vi "SPI_Example_Host.vi"() -> ()   [LabVIEW 2012]
uses:
  SPI Host API/Controls/FPGA SPI_SPI Configuration Cluster.ctl
  <vilib>/FPGAPlugInAG/sbRIO-9636/niLvFpga_Open_sbRIO-9636.vi
  <vilib>/FPGAPlugInAG/sbRIO-9636/niLvFpga_Close_sbRIO-9636.vi
  <vilib>/rvi/interface/nirviOpenFPGA/nirviOpenFPGA.xnode
  SPI Host API/Controls/FPGA SPI_FPGA Ref.ctl
  FPGA Bitfiles/NIARC_FPGATarget_SPIFPGATopLevelM_H-QxMroaqT4.lvbitx
  FPGA/SPI_FPGA_Top_Level_Main.vi
  <vilib>/rvi/interface/nirviCloseFPGA/nirviCloseFPGA.xnode
panel:
  out "Byte count":i32
  in  "Perform Startup":bool
  out "array":u8[](array[numeric]) format="%.0x"
  out "error out":errorcluster
  in  "stop":bool
  in  "Write Data":u8[](array[numeric]) format="%.0x"
  in  "Configuration Cluster":T1={"CS"=1, "Clock Rate (Hz)"=50000.0, "Clock Mode"=0, "CS Active State"=FALSE} {"CS" items=["0"=1, "1"=2, "2"=4, "3"=8, "4"=16, "5"=32, "6"=64, "7"=128]; "Clock Mode" items=["0", "1", "2", "3"]}
  in  "Total Bits":u16=8
  out "Read Data":u8[](array[numeric])
  in  "Write":bool
  # "Configure SPI"
  # "Write SPI"
  # "Control and Status"
  # "Read SPI"
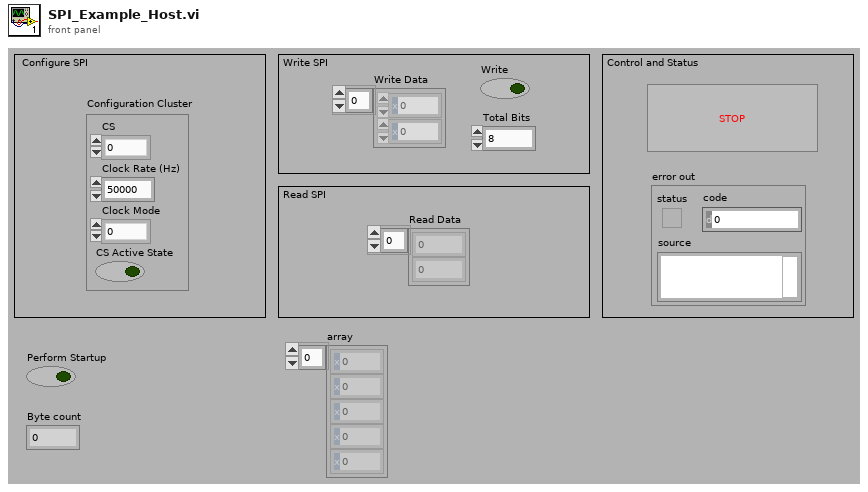
[diagram p1: front panel]
types:
  T1 = typedef "FPGA SPI_SPI Configuration Cluster.ctl" = cluster{"CS":u8, "Clock Rate (Hz)":dbl, "Clock Mode":u8, "CS Active State":bool}
  T2 = typedef "FPGA SPI_FPGA Ref.ctl" = refnum<k20>
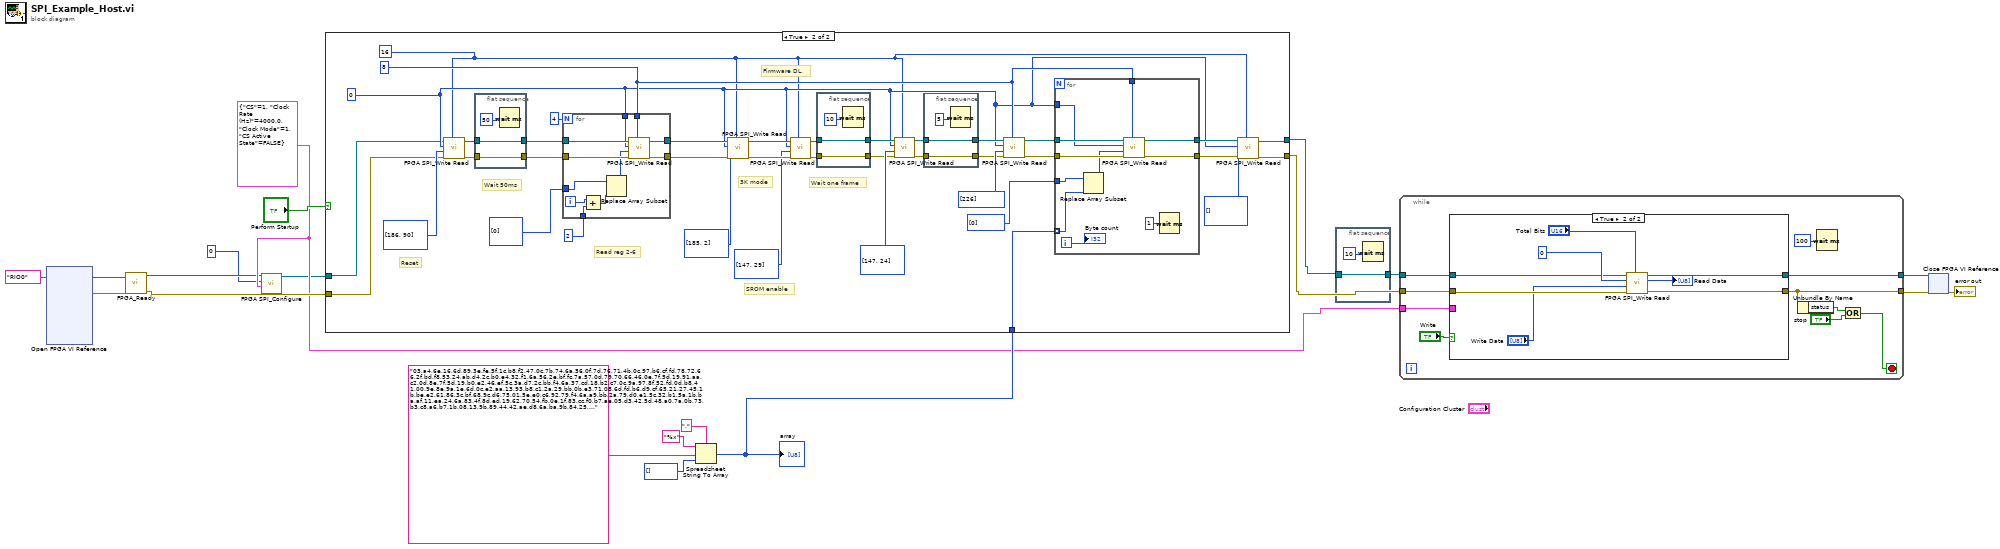
[diagram p0: block diagram]
diagram:
  w4 = T1 {"CS"=1, "Clock Rate (Hz)"=4000.0, "Clock Mode"=1, "CS Active State"=FALSE} ("Configuration Cluster")
  n1 = xnode "Open FPGA VI Reference"("resource name"=tag "RIO0") -> ("FPGA VI Reference Out"=w20:T2, "error out"=w19:errorcluster)  [unwired: 1 in]
  n2 = call "FPGA_Ready.vi"("Error In"=w19, "FPGA VI Reference In"=w20) -> ("Error Out"=w14:errorcluster, "FPGA VI Reference Out"=w3:T2)  [unwired: 7 out]
  n3 = call "FPGA SPI_Configure.vi"("Configuration Cluster"=w4, "Port"=u8 0, "FPGA VI Reference"=w3) -> ("FPGA VI Reference Out"=w2:T2)  [unwired: 1 in, 7 out]
  n4 = Spreadsheet String To Array(delimiter (Tab)=",", format string="%x", spreadsheet string="03,a4,6e,16,6d,89,3e,fe,5f,1c,b8,f2,47,0c,7b,74,6a,56,0f,7d,76,71,4b,0c,97,b6,cf,fd,78,72,66,2f,bd,f8,53,24,ab,d4,2c,b0,e4,32,f1,6a,56,2e,bf,fc,7a,57,0d,79,70,66,46,0e,7f,5d,19,91,aa,c2,0d,8e,7f,5d,19,b0,e2,46,ef,5c,3a,d7,2c,bb,f4,6a,37,cd,18,b2,c7,0c,9a,97,8f,52,fd,0d,b8,41,00,9e,8e,9a,1e,6d,0c,e2,aa,13,93,b8,c1,2a,29,bb,0b,e3,71,08,6d,fd,b6,d9,cf,65,21,27,45,1b,be,e2,61,86,3c,bf,68,9c,d6,75,01,5e,e0,c6,92,79,f4,6a,a9,bb,2a,79,d0,e1,5c,32,b1,5a,1b,ba,af,11,ea,24,6a,83,4f,8d,ed,19,62,70,54,fb,0e,1f,83,cc,f0,b7,ae,05,d3,42,5d,48,a0,7a,0b,73,b3,c8,a6,b7,1b,08,13,9b,89,44,42,ae,d8,6a,ba,9b,84,25,8b,a4,5e,0b,85,b0,8f,8d,80,9c,d1,52,c7,cb,ff,8d,8b,dd,87,f2,63,ca,e7,4f,4a,57,3c,df,af,cb,5c,bb,39,0b,01,9c,79,22,15,b8,a0,d3,72,02,35,20,40,e0,17,de,89,88,ce,e9,2b,75,ba,a0,96,24,1e,71,b5,15,00,61,e0,5c,93,4e,ea,53,d0,fc,ef,ae,2b,eb,8f,c7,69,68,c7,fc,1a,1f,41,0d,d0,c1,03,af,c9,fd,e4,21,43,c4,ef,c2,dd,7b,73,bc,ca,f4,a5,2e,83,90,1f,78,41,c3,13,8e,95,0a,57,df,0a,87,40,2b,d9,ba,56,59,9d,2c,b2,b8,b3,fb,77,78,3a,ef,bf,2d,c8,b9,94,62,47,92,98,42,23,07,d9,39,46,5e,6f,e0,46,14,0e,3d,74,40,21,b4,67,05,a8,e2,12,93,41,c2,80,b9,56,4b,f9,5a,15,9c,37,c4,4b,05,ad,5a,af,a1,3e,e4,6e,c5,91,b6,75,7d,1b,e4,c5,4d,28,6b,e9,ad,20,8b,64,91,57,4f,df,9a,97,7e,be,8e,d6,d6,3b,17,f9,19,28,b2,2e,8f,26,b4,9b,e5,de,0f,8d,0a,9a,9d,1b,de,6f,cb,84,ba,26,d0,12,ef,30,38,43,ac,b7,a7,ef,09,7c,52,27,fc,2e,ab,50,a0,21,40,e7,c1,5f,02,41,84,a8,54,a8,2e,37,6f,d8,b1,a4,d0,75,ef,31,ca,54,1e,33,ad,19,a1,94,bc,1b,34,6c,fb,5f,cc,45,76,c8,96,ce,1c,3a,0e,77,ed,d8,d2,96,ac,77,30,e1,ef,b0,33,f0,6e,3d,ce,5e,6d,de,8a,dc,9b,91,63,2a,95,20,0d,fd,78,ba,cb,15,43,c9,20,96,83,06,d9,11,f3,e2,13,cf,9c,91,7f,33,46,a7,e2,d3,75,ff,4f,0c,0c,af,cd,a6,9c,a6,73,e2,6d,17,16,b5,99,80,35,d9,61,f3,48,23,ff,ae,53,89,fa,55,1c,37,a5,e8,62,12,b2,22,04,ed,42,b6,65,c4,41,42,72,ca,7e,5e,2f,69,46,ef,bd,7e,df,35,1e,5b,77,af,8d,39,f8,a7,d8,31,00,d3,85,66,d5,cd,59,d6,5e,9f,b2,3f,09,d1,c4,5b,74,62,d3,30,35,f3,e3,7d,7f,ab,38,c2,33,42,d0,67,d0,f4,cf,97,ec,35,31,fe,94,9c,a1,66,91,c8,05,45,19,85,0f,4a,b0,3a,20,44,a4,6b,33,0c,a6,b4,4c,46,30,15,2d,bb,04,3c,9d,48,f6,84,9a,62,07,e9,6c,8f,de,29,28,5a,17,ec,56,f3,c4,e0,86,2f,b5,1c,8f,aa,c6,c0,cf,0d,cf,1d,4f,b2,bf,26,5c,7c,8d,d3,e4,56,d1,e8,90,94,6a,ba,27,ba,f7,ba,39,c8,08,03,25,7f,16,8f,61,bf,df,45,88,7d,90,80,55,58,72,4f,f8,d0,94,bb,55,2a,47,4f,aa,87,2d,d4,e7,af,08,33,c9,ec,0b,5b,b8,53,27,2e,fb,ad,69,b6,53,64,48,13,41,f8,02,06,6f,b8,cc,64,ec,65,65,7e,df,3f,1e,e1,ee,de,3c,1a,e8,0f,f0,2c,ea,6e,52,77,34,41,a1,cc,72,8f,6e,9c,3b,8d,39,df,d4,08,24,ba,36,c7,09,f2,f1,a2,d1,e0,a3,6a,5c,c7,b2,0d,1c,fb,5f,c8,86,d8,3e,1c,b7,1f,2d,d8,f2,cd,52,eb,de,50,14,b7,c7,a2,8b,78,70,11,87,1a,c5,b8,e5,5e,a5,c9,94,22,66,7b,8b,74,ab,85,28,95,90,6e,07,dd,79,57,b3,75,c8,18,67,39,06,21,55,ba,ba,da,f9,3b,e9,5d,c9,1f,6f,61,3b,c2,7e,3d,07,a6,84,91,b7,63,7e,5f,fc,d1,7d,08,dd,79,07,e1,9e,11,25,e8,10,05,66,fa,ca,c3,41,01,27,54,d2,46,ae,e3,ff,43,ae,8d,0e,31,13,1f,95,79,82,86,7e,fb,d4,17,57,b8,25,e7,1d,18,8f,06,1a,e5,ef,55,28,72,42,ae,df,9e,bb,14,ab,d8,36,4f,46,4b,35,92,64,6d,bb,60,c2,0b,6f,57,5e,3a,8f,3d,cb,e5,da,6c,5c,85,8f,9d,a6,7e,1e,49,1a,cc,c9,ec,04,ab,35,f2,9b,e7,b3,52,b1,1c,c1,fe,5c,0b,f5,72,0b,ec,8e,cd,67,98,bf,a5,28,ca,48,9b,60,1c,ee,00,de,01,bc,a4,02,d2,19,b6,05,d6,52,78,db,20,bd,3f,95,97,b1,59,3d,9d,83,c2,fd,23,a5,fd,d8,20,92,27,ee,3c,e9,5a,61,11,e1,31,b4,4c,b4,a9,e2,6d,2e,ae,5f,37,8e,07,fd,ed,85,07,79,43,7e,fa,d6,03,e8,5b,65,2a,e4,f9,36,9e,ff,53,6d,51,50,61,72,18,cd,3d,e4,b6,27,10,4a,dd,fd,a3,36,67,ac,c7,85,1c,d3,e7,17,74,e2,8e,ee,a6,f4,b6,86,24,cf,40,df,35,08,0f,55,dd,51,e9,7c,39,78,5c,df,20,2a,eb,ed,35,10,26,98,77,69,4e,51,7a,b2,9f,1d,bc,06,cd,cf,4d,b9,fa,b7,af,6a,07,0c,96,42,57,6c,3d,a5,fe,91,e3,76,9f,dd,3c,83,25,ab,24,89,47,7c,ba,d7,7d,72,90,80,b0,03,a4,ef,04,0a,9e,5a,14,1c,ab,75,47,05,cb,a2,97,0d,6a,a5,7c,a4,40,90,e2,6c,fa,d4,bd,69,d0,06,53,67,fa,e7,cc,06,42,45,be,bd,6f,3e,48,70,f5,2b,83,c7,ba,54,9c,ab,54,1f,81,e2,11,82,51,02,51,63,13,86,38,b1,56,0c,4d,68,f3,53,1d,fb,e3,15,e8,42,f3,27,9b,a5,4a,86,90,e1,17,dc,99,e2,5c,79,c6,5f,7e,33,c0,41,b6,9e,fc,10,8a,f4,fd,e9,d2,52,53,54,89,04,bd,69,d2,54,32,96,ec,44,08,c3,86,10,d1,3e,32,b5,4f,52,49,58,49,f2,8d,83,89,f3,24,83,65,72,53,af,2d,90,61,99,92,31,75,93,46,e5,d3,48,11,01,c9,10,98,66,86,79,19,73,7d,da,a1,b0,41,9e,cd,dc,c2,66,86,dd,b8,c9,e3,e7,80,96,f5,38,72,a5,da,e5,38,13,57,2b,bd,32,c7,44,e0,e3,2d,ed,54,40,74,9d,02,55,38,45,89,6f,14,40,f6,7b,41,1e,04,db,a4,d9,f3,90,ae,10,c9,c3,72,5d,0d,01,51,f1,d1,96,43,c6,1a,98,3d,bd,cd,df,44,82,d0,17,a2,9e,6c,0c,2f,46,eb,d8,4a,ce,fe,be,cd,f9,d4,e3,36,f3,d8,1c,00,24,f2,ac,03,11,b6,18,8f,9c,ba,f6,4f,fd,78,72,83,bf,3e,5c,24,f9,4d,ea,85,74,25,e3,46,7b,5e,fe,bd,bf,5e,68,51,e5,53,85,9a,03,4c,09,f0,6b,c2,97,fc,cc,96,2c,af,f7,8c,26,d8,c7,fc,da,1f,0e,0f,39,1a,b2,0a,98,1a,15,dc,3e,4b,9e,9d,40,3e,71,5b,66,c3,88,f8,57,14,06,c7,2c,cd,31,8e,1e,88,79,9f,33,94,ea,21,08,0d,35,7d,a2,57,46,e3,0f,b9,a9,bc,d2,06,b8,fa,f9,b0,f3,c3,8a,38,82,06,7f,d9,ce,92,a2,9e,fc,2a,c8,51,b7,7d,db,47,37,af,8b,b8,6d,70,21,02,63,5e,bd,38,f1,e1,9f,e3,e2,79,3b,42,05,e2,c6,13,7a,e2,91,73,e2,79,8b,2f,7f,88,02,06,4e,b8,66,b8,c0,c4,3b,1c,3e,96,0f,bb,7f,e8,85,5b,b2,f6,a7,48,5b,95,83,57,e0,e8,22,67,07,3c,27,65,66,e8,84,ab,ea,f5,b5,00,ec,a4,a3,e8,25,77,d1,81,9c,87,d3,1a,31,58,a4,0a,a8,71,9c,52,88,4d,50,ff,db,41,81,04,c3,84,aa,72,79,2f,9b,2d,2f,1c,a5,6b,68,9b,3b,6b,1c,67,eb,42,e0,e3,2c,7b,52,8e,c1,7e,d8,ab,02,46,d1,83,38,1a,18,ad,90,7f,db,22,c1,80,ea,f7,67,1d,a7,b2,40,db,c3,c4,d5,8b,49,f8,dc,25,80,7e,fa,64,ac,36,4d,74,6f,3e,57,23,b4,49,7c,6f,3e,7c,a7,34,b7,6b,66,f8,d1,69,6d,83,c5,8a,e2,42,3f,8b,5e,5a,d5,cd,47,64,eb,4e,ef,62,19,37,d3,8e,68,51,4a,96,bb,5b,a0,34,d8,b4,f4,b0,99,53,b1,70,c3,1d,6e,2b,03,76,c9,00,0b,10,ca,b7,f3,be,4b,e2,b4,6c,4a,9f,59,39,30,c7,c3,88,38,63,c4,cf,d1,fd,f0,6d,fe,68,92,98,11,7d,90,0c,64,23,e8,25,77,d1,81,75,a4,f4,35,6f,e4,9c,7a,48,d0,de,37,42,f8,5b,e9,16,ba,16,4b,7c,db,2c,0e,a0,bc,5c,82,71,a0,9d,3a,0a,7e,d0,dc,93,79,f6,78,b5,89,d9,70,5d,e0,9d,e7,ea,ee,88,52,18,11,7d,f1,ce,c1,69,8d,3f,ea,51,c1,49,b1,c4,a6,f0,dc,bd,61,b7,2c,85,4a,cb,dd,96,50,8b,68,f7,7e,b9,1c,19,fb,5c,79,f8,7d,e9,f3,0e,c7,6e,1c,67,b4,b7,4a,c5,be,3c,8c,94,36,02,8f,81,57,e7,4b,d6,2b,10,be,3c,97,bb,41,88,6f,13,e6,27,13,4b,d5,44,a9,d9,2d,cd,51,91,03,14,d5,6b,3d,b5,98,f0,09,aa,42,8e,82,e8,f1,36,ec,b5,48,5f,9f,ca,16,5a,3f,4d,bb,a6,d4,08,1a,fb,e5,eb,40,04,e8,40,84,c4,8e,74,ae,47,4d,fc,b5,91,e2,33,f2,f7,ae,cd,10,47,b1,4b,e2,a2,8d,7c,2c,32,6f,dd,c4,c2,f1,09,56,2d,1e,9d,7d,67,32,61,7f,12,e4,3f,fa,e2,7d,7b,d4,67,4e,7f,14,6a,6c,8e,74,9b,bc,3d,c4,70,c4,37,d5,60,e0,87,bd,b8,1a,75,9d,7a,80,c1,a9,1f,ad,7b,27,e5,4c,b0,06,d0,fb,1c,5a,eb,bd,2e,96,49,13,43,06,8b,cb,6a,f0,5d,56,6c,4e,18,26,d4,c8,53,48,70,e2,0f,9c,a1,35,01,96,c7,0b,c9,4b,d3,19,e8,5a,75,ad,c8,52,ce,3c,2e,fd,5f,04,cf,9e,d6,33,db,08,34,ba,34,9b,f4,25,aa,7f,52,37,4f,8b,94,95,94,2d,88,10,d1,05,07,cf,d4,04,db,95,be,36,d0,1c,1c,a4,85,0a,02,80,de,b1,1b,56,af,51,22,a7,a4,4a,2c,2f,17,7c,13,4c,36,ad,90,8c,ea,d4,58,3a,ca,ea,1d,5c,6c,93,ad,59,ed,b1,17,a4,22,95,67,be,bb,25,af,65,c8,e5,90,e1,17,dc,7a,47,e9,8f,c3,c3,5a,dc,20,20,4a,09,fc,39,51,29,31,fb,a0,0a,61,08,9b,b9,b3,6c,95,c5,94,00,66,f1,b9,79,90,7f,95,5f,55,e1,13,6b,87,a8,62,21,98,f2,57,19,92,10,b3,24,81,12,21,ff,d6,f9,73,71,c2,62,09,31,eb,e0,7a,35,60,8d,c9,b1,e5,a7,8b,ca,bc,2d,fa,63,c7,68,1d,19,b5,61,78,d0,8b,db,c0,39,22,55,6a,28,c2,52,1e,6b,f7,1d,b6,fa,4f,cf,27,7c,af,7f,0c,96,ba,ce,2a,54,59,5b,20,fb,42,87,44,d9,2e,10,43,ab,58,92,b6,8d,78,f3,a3,de,0e,07,75,68,52,26,3f,3d,ec,d0,36,df,1a,16,88,5f,bd,1c,4d,9e,27,4c,12,07,0d,2b,b1,dc,00,45,54,3d,fc,cf,fa,c9,06,4b,08,64,ac,8d,17,4d,df,83,24,fb,f6,9e,5f,f9,0f,8d,07,18,b1,b2,37,d2,66,9c,82,09,75,52,5b,19,74,59,a3,64,6d,17,93,3a,13,d2,da,97,a4,2b,55,7a,32,f9,2f,9b,aa,87,6d,ce,1d,07,9a,52,fa,40,c5,20,43,cc,a8,c3,84,2c,44,8b,44,88,62,e7,68,4c,2a,69,a7,cf,6f,4d,06,ed,8a,8f,9a,62,ca,ed,a5,57,18,86,9d,e8,7c,14,eb,71,eb,c0,f4,3a,98,11,01,c0,a3,53,af,20,7e,de,22,5c,1f,60,8b,b7,5f,74,76,d0,87,fa,11,d3,a5,ba,5c,82,e1,52,54,6b,69,eb,31,43,01,1a,55,7f,dc,2f,d8,01,26,6f,1c,2d,72,7b,c8,93,99,2a,08,a8,6f,b4,28,40,8a,8a,4e,d5,3b,39,45,a8,e4,e7,73,8f,00,64,d3,c7,87,de,43,82,2c,e8,57,17,29,ce,b8,47,d6,08,79,d7,c4,e9,23,43,9d,b8,cb,78,08,32,f1,ec,84,80,1e,b9,29,12,0c,29,cc,9c,d0,10,a7,d6,8a,e9,f6,fa,8d,7e,95,2e,57,cf,8e,38,6b,35,f0,bc,a6,4e,13,7b,41,19,15,5d,99,bd,22,40,6a,07,2d,d5,d6,ff,1d,7b,a6,c4,aa,77,44,78,2f,55,9f,7d,53,f0,2b,2b,ba,36,c2,f8,6d,f0,2b,bb,6b,97,05,b4,4a,c2,86,62,b8,76,e7,bb,df,9c,5a,70,19,95,59,15,cf,a6,a9,7a,24,4c,c6,65,b9,da,17,6f,2b,55,07,32,72,d1,ee,9c,3a,51,98,36,37,f8,61,fc,91,bc,cb,34,d8,43,a0,7a,ea,c4,8a,64,4d,e0,03,93,fb,b4,d8,11,21,11,66,97,b9,ba,81,29,c2,8f,8c,14,18,22,94,c4,b0,f1,10,c4,8b,5d,8d,7f,14,af,46,19,36,a4,36,22,18,18,e3,ab,2c,91,03,f7,c5,f5,f5,59,c2,d2,f7,c7,64,54,76,fb,71,70,e8,b2,44,a1,2d,59,17,02,d6,6f,7a,eb,e0,53,81,f6,5e,7f,37,d4,52,13,04,44,d5,c8,d3,dd,6f,d5,fb,71,20,e3,0d,0c,47,25,a1,41,d2,c7,e5,c9,d9,27,a5,38,e4,30,bb,86,07,84,ef,24,9f,f9,52,74,d2,50,73,c4,27,73,3b,8d,9c,a6,f6,4b,25,91,c5,9e,1e,b2,78,0c,23,80,dd,a3,21,f5,a9,9e,00,16,19,bc,d9,55,09,90,a2,c6,ef,3d,f8,72,66,2f,dc,3a,f6,4f,fd,59,30,e2,27,cc,fb,55,09,71,41,e1,21,a1,a1,c0,e3,25,a9,d0,22,c6,ef,5c,1b,b4,ea,56,2e,bf,fc,5b,34,cb,14,8b,94,aa,b7,ec,5a,36,cf,1c,ba,f6,4d,db,35,f3", array type (2D Dbl)=u8[] []) -> (array=w8:u8[])
  "array" <- w8
  n5 = case shown="True" "Perform Startup" {
    tunnel: w2 -> [w22 w24]
    tunnel: w14 -> [w21 w23]
    tunnel: [w22 w29] -> w6
    tunnel: [w21 w28] -> w7
    tunnel: w8 -> [_ w40]
    frame False {
    }
    frame True {
      w32 = u16 8 ("Total Bits")
      w26 = u16 16 ("Total Bits")
      w27 = u8 0 ("Port")
      # "Wait one frame"
      # "SROM enable"
      # "3K mode"
      # "Firmware DL."
      # "Read reg 2-6"
      # "Wait 50ms"
      # "Reset"
      n6 = call "FPGA SPI_Write Read.vi"("Total Bits"=w26, "error in"=w23, "Write Data"=u8[] [186, 90], "Port"=w27, "FPGA VI Reference"=w24) -> ("error out"=w58:errorcluster, "FPGA VI Reference Out"=w59:T2)  [unwired: 5 out]
      n7 = flat-sequence {
        tunnel: w59 -> [w90]
        tunnel: w58 -> [w89]
        tunnel: [w90] -> w57
        tunnel: [w89] -> w56
        frame #0 {
          n8 = Wait (ms)(milliseconds to wait=u32 50) -> ()  [unwired: 1 out]
        }
      }
      n9 = for {
        N: 4 -> [_]
        tunnel: w57 -> [w88]
        tunnel: w27 -> [w87]
        tunnel: [w86] -> w51
        tunnel: [w85] -> w52
        tunnel: w56 -> [w84]
        tunnel: u8[] [0] ("Write Data") -> [w83]
        tunnel: 2 ("y") -> [w79]
        tunnel: w32 -> [w78]
        i -> [w80]
        n10 = Add(x=w80, y=w79) -> (x+y=w81:i32)
        n11 = Replace Array Subset(array=w83, new element=w81) -> (w82:u8[])  [unwired: 1 in]
        n12 = call "FPGA SPI_Write Read.vi"("Total Bits"=w78, "error in"=w84, "Write Data"=w82, "Port"=w87, "FPGA VI Reference"=w88) -> ("error out"=w85:errorcluster, "FPGA VI Reference Out"=w86:T2)  [unwired: 5 out]
      }
      n13 = call "FPGA SPI_Write Read.vi"("Total Bits"=w26, "error in"=w52, "Write Data"=u8[] [185, 2], "Port"=w27, "FPGA VI Reference"=w51) -> ("error out"=w49:errorcluster, "FPGA VI Reference Out"=w48:T2)  [unwired: 5 out]
      n14 = call "FPGA SPI_Write Read.vi"("Total Bits"=w26, "error in"=w49, "Write Data"=u8[] [147, 29], "Port"=w27, "FPGA VI Reference"=w48) -> ("error out"=w45:errorcluster, "FPGA VI Reference Out"=w46:T2)  [unwired: 5 out]
      n15 = flat-sequence {
        tunnel: w46 -> [w76]
        tunnel: w45 -> [w75]
        tunnel: [w76] -> w42
        tunnel: [w75] -> w43
        frame #0 {
          n16 = Wait (ms)(milliseconds to wait=u32 10) -> ()  [unwired: 1 out]
        }
      }
      n17 = call "FPGA SPI_Write Read.vi"("Total Bits"=w26, "error in"=w43, "Write Data"=u8[] [147, 24], "Port"=w27, "FPGA VI Reference"=w42) -> ("error out"=w36:errorcluster, "FPGA VI Reference Out"=w37:T2)  [unwired: 5 out]
      n18 = flat-sequence {
        tunnel: w37 -> [w62]
        tunnel: w36 -> [w61]
        tunnel: [w62] -> w35
        tunnel: [w61] -> w34
        frame #0 {
          n19 = Wait (ms)(milliseconds to wait=u32 5) -> ()  [unwired: 1 out]
        }
      }
      n20 = call "FPGA SPI_Write Read.vi"("Total Bits"=w32, "error in"=w34, "Write Data"=u8[] [226], "Port"=w27, "FPGA VI Reference"=w35) -> ("error out"=w38:errorcluster, "FPGA VI Reference Out"=w39:T2)  [unwired: 5 out]
      n21 = for {
        tunnel: w40 -> [w68] mode=indexing
        tunnel: w39 -> [w74]
        tunnel: w38 -> [w73]
        tunnel: [w72] -> w31
        tunnel: [w71] -> w30
        tunnel: u8[] [0] -> [w69]
        tunnel: w32 -> [w66]
        tunnel: w27 -> [w65]
        i -> [w64]
        n22 = Replace Array Subset(array=w69, new element=w68) -> (w67:u8[])  [unwired: 1 in]
        n23 = call "FPGA SPI_Write Read.vi"("Total Bits"=w66, "error in"=w73, "Write Data"=w67, "Port"=w65, "FPGA VI Reference"=w74) -> ("error out"=w71:errorcluster, "FPGA VI Reference Out"=w72:T2)  [unwired: 5 out]
        n24 = Wait (ms)(milliseconds to wait=u32 1) -> ()  [unwired: 1 out]
        "Byte count" <- w64
      }
      n25 = call "FPGA SPI_Write Read.vi"("Total Bits"=w26, "error in"=w30, "Write Data"=u8[] [], "Port"=w27, "FPGA VI Reference"=w31) -> ("error out"=w28:errorcluster, "FPGA VI Reference Out"=w29:T2)  [unwired: 5 out]
    }
  }
  n26 = flat-sequence {
    tunnel: w6 -> [w92]
    tunnel: [w92] -> w5
    frame #0 {
      n27 = Wait (ms)(milliseconds to wait=u32 10) -> ()  [unwired: 1 out]
    }
  }
  n28 = while {
    tunnel: w5 -> [w103]
    tunnel: w7 -> [w102]
    tunnel: [w100] -> w18
    tunnel: [w99] -> w17
    tunnel: w4 -> [w94]
    stop <- w95 stop-if-true
    n29 = case shown="True" "Write" {
      tunnel: w103 -> [w105 w108]
      tunnel: w102 -> [w104 w107]
      tunnel: [w104 w113] -> w99
      tunnel: [w105 w112] -> w100
      tunnel: w94 -> [_ _]
      frame False {
      }
      frame True {
        n30 = call "FPGA SPI_Write Read.vi"("Total Bits"="Total Bits", "error in"=w107, "Write Data"="Write Data", "Port"=u8 0, "FPGA VI Reference"=w108) -> ("error out"=w113:errorcluster, "Read Data"=→"Read Data":u8[], "FPGA VI Reference Out"=w112:T2)  [unwired: 4 out]
      }
    }
    n31 = Unbundle By Name(w99) -> ("status"=w97:bool)
    n32 = Wait (ms)(milliseconds to wait=u32 100) -> ()  [unwired: 1 out]
    n33 = Compound Arithmetic op=OR(w97, "stop") -> (w95:bool)
  }
  n34 = xnode "Close FPGA VI Reference"("FPGA VI Reference In"=w18, "error in"=w17) -> ("error out"=→"error out":errorcluster)
